vi "drawString.vi"(0 "reference":refnum<class "StateTransitionEdge.lvclass">, 1 "graphics":refnum<class "Graphics.lvclass">, 2 "p1":T1 {"y" format="%.2f"; "x" format="%.2f"}, 3 "p2":T1 {"y" format="%.2f"; "x" format="%.2f"}, 4 "text":string, 5 "error in (no error)":errorcluster, 6 "Offset":T1 {"y" format="%.2f"; "x" format="%.2f"}, 7 "center":bool) -> (14 "reference out":refnum<class "StateTransitionEdge.lvclass">, 19 "error out":errorcluster)   [LabVIEW 2014, in "StateTransitionEdge.lvclass"]
doc: "\"public static void drawString(Graphics2D g2,"
uses:
  <resource>/Framework/Providers/Open_GDS/UML/StateTransitionEdge_class/StateTransitionEdge.lvclass
  <resource>/Framework/Providers/Open_GDS/UML/Graphics_class/Graphics.lvclass
  <resource>/Framework/Providers/Open_GDS/UML/General/Point/Point Point2D.ctl
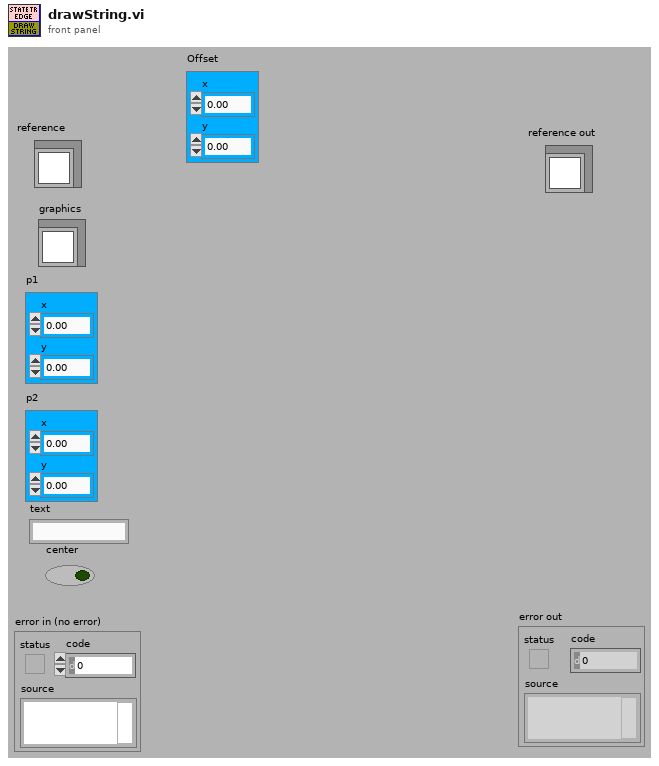
[diagram p1: front panel]
types:
  T1 = typedef "Point Point2D.ctl" = cluster{"x":dbl, "y":dbl}
  T2 = typedef "Rectangle Rectangle2D.ctl" = cluster{"x":dbl, "y":dbl, "width":dbl, "height":dbl}
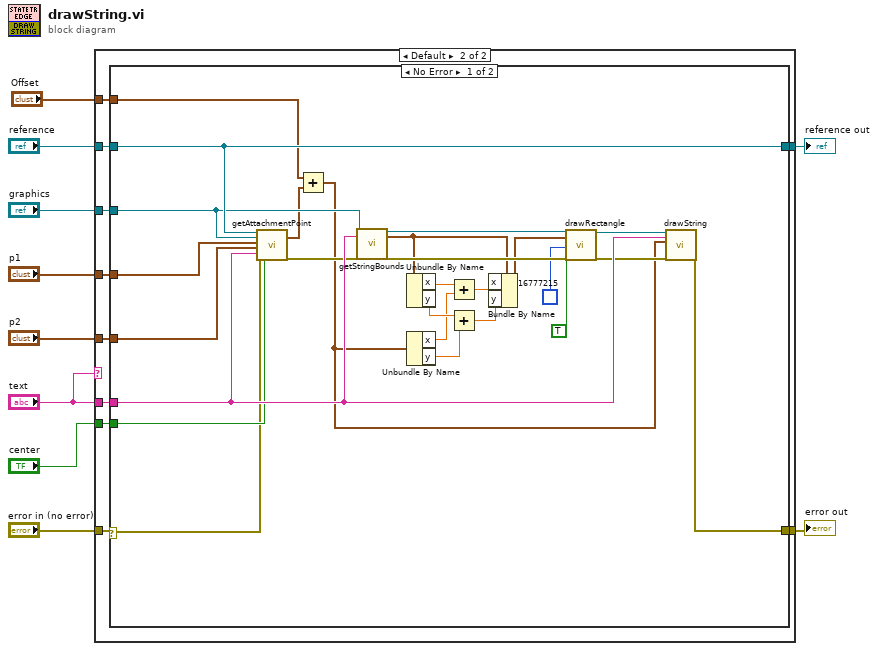
[diagram p0: block diagram]
diagram:
  n1 = case shown="Default" "text" {
    tunnel: "reference" -> [w12 w22]
    tunnel: [w11 w21] -> w9
    tunnel: [w12 w20] -> w8
    tunnel: "error in (no error)" -> [w11 w19]
    tunnel: "graphics" -> [_ w18]
    tunnel: "text" -> [_ w17]
    tunnel: "p1" -> [_ w16]
    tunnel: "p2" -> [_ w15]
    tunnel: "center" -> [_ w14]
    tunnel: "Offset" -> [_ w13]
    frame "" {
    }
    frame Default {
      n2 = case shown="No Error" w19 {
        selector: w19 -> [w26 w49]
        tunnel: w22 -> [w48 w50]
        tunnel: [w47 w49] -> w21
        tunnel: [w48 w50] -> w20
        tunnel: w18 -> [w46 _]
        tunnel: w17 -> [w45 _]
        tunnel: w16 -> [w44 _]
        tunnel: w15 -> [w43 _]
        tunnel: w14 -> [w42 _]
        tunnel: w13 -> [w25 _]
        frame No Error {
          n3 = call-dynamic "getAttachmentPoint.vi"("reference"=w48, "graphics"=w46, "p1"=w44, "p2"=w43, "text"=w45, "error in (no error)"=w26, "center"=w42) -> ("attachPoint"=w24:T1, "error out"=w41:errorcluster)  [unwired: 10 in, 1 out]
          n4 = Add(x=w25, y=w24) -> (x+y=w23:T1)
          n5 = call-dynamic "getStringBounds.vi"("reference"=w46, "text"=w45, "error in (no error)"=w41) -> ("reference out"=w39:refnum<class "Graphics.lvclass">, "bounds"=w34:T2, "error out"=w40:errorcluster)  [unwired: 14 in]
          n6 = Unbundle By Name(w34) -> ("x"=w33:dbl, "y"=w31:dbl)
          n7 = Unbundle By Name(w23) -> ("x"=w28:dbl, "y"=w29:dbl)
          n8 = Add(x=w33, y=w28) -> (x+y=w32:dbl)
          n9 = Add(x=w31, y=w29) -> (x+y=w30:dbl)
          n10 = Bundle By Name(cluster=w34, "x"=w32, "y"=w30) -> (w35:T2)
          n11 = call <resource>:"drawRectangle.vi"("reference"=w39, "rectangle"=w35, "color(if not used=default color)"=u32 16777215, "fill?(F)"=TRUE, "error in (no error)"=w40) -> ("reference out"=w37:refnum<class "Graphics.lvclass">, "error out"=w36:errorcluster)  [unwired: 2 in, 11 out]
          n12 = call-dynamic "drawString.vi"("reference"=w37, "text"=w45, "textPos"=w23, "error in (no error)"=w36) -> ("error out"=w47:errorcluster)  [unwired: 14 in, 1 out]
        }
        frame Error {
        }
      }
    }
  }
  "reference out" <- w8
  "error out" <- w9
